vi "getLoadCellSignalLONG.vi"(11 "DAQmx Physical Channel":tag="Dev2/ai0:31") -> (3 "load cell\nsignal":dbl[](array[numeric]))   [LabVIEW 2017]
doc: "Measures the voltage output by the load cell across all the selected channels.\nMultiple samples are taken, filtered and then averaged. \nDuration of measurement is hard-wired."
uses:
  <vilib>/Analysis/3filter.llb/Filter Passband Type.ctl
  <vilib>/DAQmx/read.llb/DAQmx Read (Analog 2D DBL NChan NSamp).vi
  <vilib>/Analysis/baseanly.llb/Mean (DBL).vi
  <vilib>/DAQmx/create/channels.llb/DAQmx Create Channel (AI-Voltage-Basic).vi
  <vilib>/DAQmx/configure/timing.llb/DAQmx Timing (Sample Clock).vi
  <vilib>/DAQmx/miscellaneous.llb/DAQmx Fill In Error Info.vi
  <vilib>/Analysis/3filter.llb/Butterworth Filter (DBL).vi
  <vilib>/Analysis/NI_AALBase.lvlib
panel:
  in  "sample mode":i32(ring)=10178 items=["Finite Samples"=10178, "Continuous Samples"=10123, "Hardware Timed Single Point"=12522]
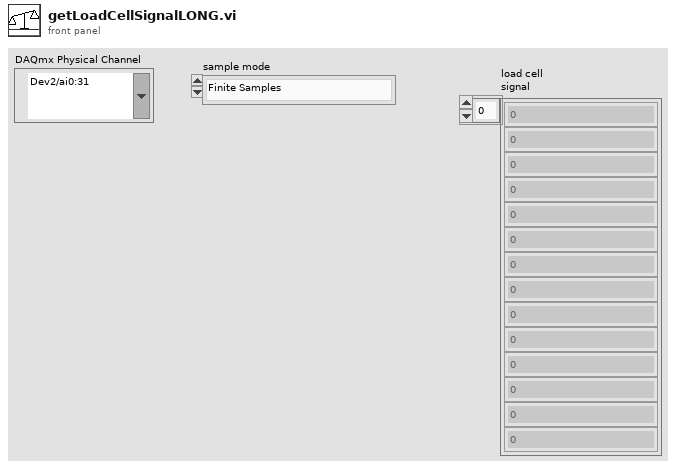
[diagram p1: front panel]
types:
  T1 = typedef "NI_AALBase.lvlib/Filter Passband Type.ctl" = enum32{"Lowpass", "Highpass", "Bandpass", "Bandstop"}
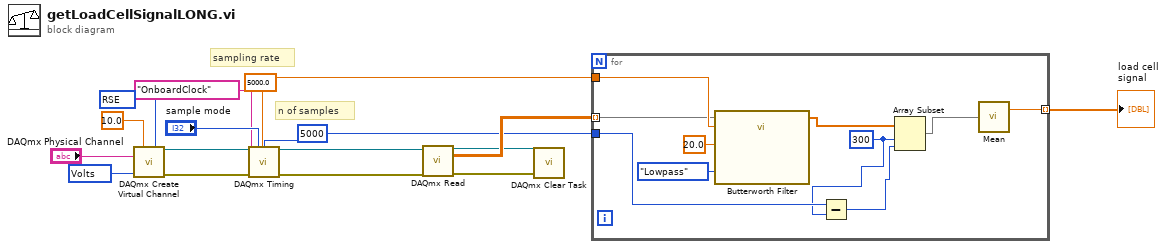
[diagram p0: block diagram]
diagram:
  w5 = 10348 items=["Volts"=10348, "From Custom Scale"=10065] ("units")
  w6 = 10083 items=["Default"=-1, "RSE"=10083, "NRSE"=10078, "Differential"=10106, "Pseudodifferential"=12529] ("input terminal configuration")
  w10 = 5000.0 ("rate")
  w1 = 5000 ("samples per channel")
  # "n of samples"
  # "sampling rate"
  n1 = call-poly <vilib>:"DAQmx Create Virtual Channel.vi"("maximum value"=10.0, "input terminal configuration"=w6, "physical channels"="DAQmx Physical Channel", "units"=w5) -> ("task out"=w16:refnum<k21>, "error out"=w13:errorcluster)  [unwired: 10 in]
  n2 = call-poly <vilib>:"DAQmx Timing.vi"("task/channels in"=w16, "sample mode"="sample mode", "samples per channel"=w1, "rate"=w10, "source"=tag "OnboardClock", "error in"=w13) -> ("task out"=w14:refnum<k21>, "error out"=w12:errorcluster)  [unwired: 8 in]
  n3 = call-poly <vilib>:"DAQmx Read.vi"("task/channels in"=w14, "error in"=w12) -> ("task out"=w8:refnum<k21>, "data"=w11:dbl[][], "error out"=w7:errorcluster)  [unwired: 11 in]
  n4 = call <vilib>:"DAQmx Clear Task.vi"("task in"=w8, "error in"=w7) -> ()  [unwired: 13 in, 1 out]
  n5 = for {
    tunnel: w11 -> [w25] mode=indexing
    tunnel: w10 -> [w26]
    tunnel: [w24] -> w2 mode=indexing
    tunnel: w1 -> [w19]
    w18 = 300 ("index")
    n6 = call-poly <vilib>:"Butterworth Filter.vi"("filter type"=Filter_Passband_Type."Lowpass", "low cutoff freq: fl"=20.0, "sampling freq: fs"=w26, "X"=w25) -> ("Filtered X"=w21:dbl[])  [unwired: 4 in, 1 out]
    n7 = Subtract(x=w19, y=w18) -> (x-y=w17:i32)
    n8 = Array Subset(array=w21, index=w18, length=w17) -> (w20:dbl[])
    n9 = call-poly <vilib>:"Mean.vi"("X"=w20) -> ("mean"=w24:dbl)  [unwired: 1 out]
  }
  "load cell\nsignal" <- w2
